vi "GUI_Bella_IP2_plasma1.vi"() -> ()   [LabVIEW 2020]
uses:
  Shared/GUI_Template/GUI_master/tcp_new_data_event.ctl
  Shared/GUI_Template/GUI_master/tcp new data cluster.ctl
  Device Drivers/FilterWheels/posTypDef.ctl
  <vilib>/vision/Image Controls.llb/IMAQ Image.ctl
panel:
  in  "GUIdevice 21":string="FW-PL1-General"
  in  "pos.Channel4::21":T1=enum."4" caption="dpm cam"
  in  "Position.Axis 1::9":dbl=0.00011 caption="DPM - Y" min=-200.0 max=200.0 format="%.3g"
  in  "Boolean":bool
  out "String":string="off"
  in  "position::20":dbl=0.049403 caption="DPM_aligncam" min=0.0 max=50.0 format="%.3g"
  in  "trigger::1":bool caption="Trigger"
  in  "trigger::2":bool caption="Trigger"
  in  "exposure::2":dbl=0.005 caption="exposure" min=3.8e-05 max=1.0 format="%.3p"
  in  "Target.X::2":dbl=200.0 caption="X" min=0.0 max=2000.0
  in  "Target.Y::2":dbl=200.0 caption="Y" min=0.0 max=2000.0
  in  "TargetSize.X::2":dbl=50.0 caption="Size X" min=2.0 max=3000.0
  in  "Color 2":u32(colorbox)=16711680 caption="Color"
  in  "TargetSize.Y::2":dbl=50.0 caption="Size Y" min=2.0 max=3000.0
  in  "Thickness 2":u8=3
  out "SideViewNorth":T2(plugin-control)
  in  "exposure::1":dbl=0.001 caption="exposure" min=3.8e-05 max=1.0 format="%.3p"
  out "DPM_Align_IP2":T2(plugin-control)
  in  "Target.X::1":dbl=838.0 caption="X" min=0.0 max=2000.0
  in  "Target.Y::1":dbl=620.0 caption="Y" min=0.0 max=2000.0
  in  "TargetSize.X::1":dbl=50.0 caption="Size X" min=2.0 max=3000.0
  in  "Color 1":u32(colorbox)=16711680 caption="Color"
  in  "TargetSize.Y::1":dbl=50.0 caption="Size Y" min=2.0 max=3000.0
  in  "Thickness 1":u8=3
  in  "GUIdevice 2":string="CAM-PL1-SideviewNorth" caption="GUIdevice 4"
  out "image::2":T2(plugin-control) caption="M1 Cam"
  out "image::1":T2(plugin-control) caption="M1 Cam"
  in  "GUIdevice 1":string="CAM-PL1-DPM_Align_IP2" caption="GUIdevice 4"
  in  "position::20":dbl=0.049403 caption="DPM_aligncam" min=0.0 max=50.0 format="%.3g"
  in  "GUIdevice 20":string="STAGE-PL1-LPmodeLong"
  in  "Position.Axis 3::8":dbl=70000.0 caption="Pico Btm \nHrz" min=-1000000.0 max=1000000.0 format="%.3g"
  in  "Position.Axis 2::9":dbl=0.00011 caption="IP2 SMF" min=0.0 max=25.0 format="%.3g"
  in  "Position.Axis 3::9":dbl=47.0 caption="Debris Shield" min=-200.0 max=200.0 format="%.3g"
  in  "GUIdevice 9":string="MCD-PL1-ESP301-1" caption="GUIdevice 4"
  in  "Position.Stage B::19":dbl=57.000013 caption="DPM - Y" min=-200.0 max=200.0 format="%.3g"
  in  "Position.Stage C::18":dbl=-36.99999 caption="DPM - Z" min=-100.0 max=100.0 format="%.3g"
  in  "Position.Stage A::18":dbl=165.499987 caption="DPM - X" min=-400.0 max=400.0 format="%.3g"
  in  "GUIdevice 19":string="MCD-PL1-NewmarkDPMY"
  in  "GUIdevice 18":string="MCD-PL1-NewmarkDPMXZ"
  in  "Position.Axis 4::8":dbl=25400.0 caption="Pico Btm \nVert" min=-100000.0 max=100000.0 format="%.3g"
  in  "Position.Axis 2::8":dbl=200.0 caption="Pico Top \nHrz" min=-100000.0 max=100000.0 format="%.3g"
  in  "Position.Axis 1::8":dbl=-8000.0 caption="Pico Top \nVert" min=-100000.0 max=100000.0 format="%.3g"
  in  "GUIdevice 8":string="MCD-PL1-picosOFI1" caption="GUIdevice 4"
  out "tcp data event":T3
  in  "stop":bool
  out "error IO 2":errorcluster
  # "Plasma 1 + M3"
  # "DPM Alignment"
  # "DPM Major Axes, Picos, Debris Shield"
  # "<----laser"
  # "Filter Wheels"
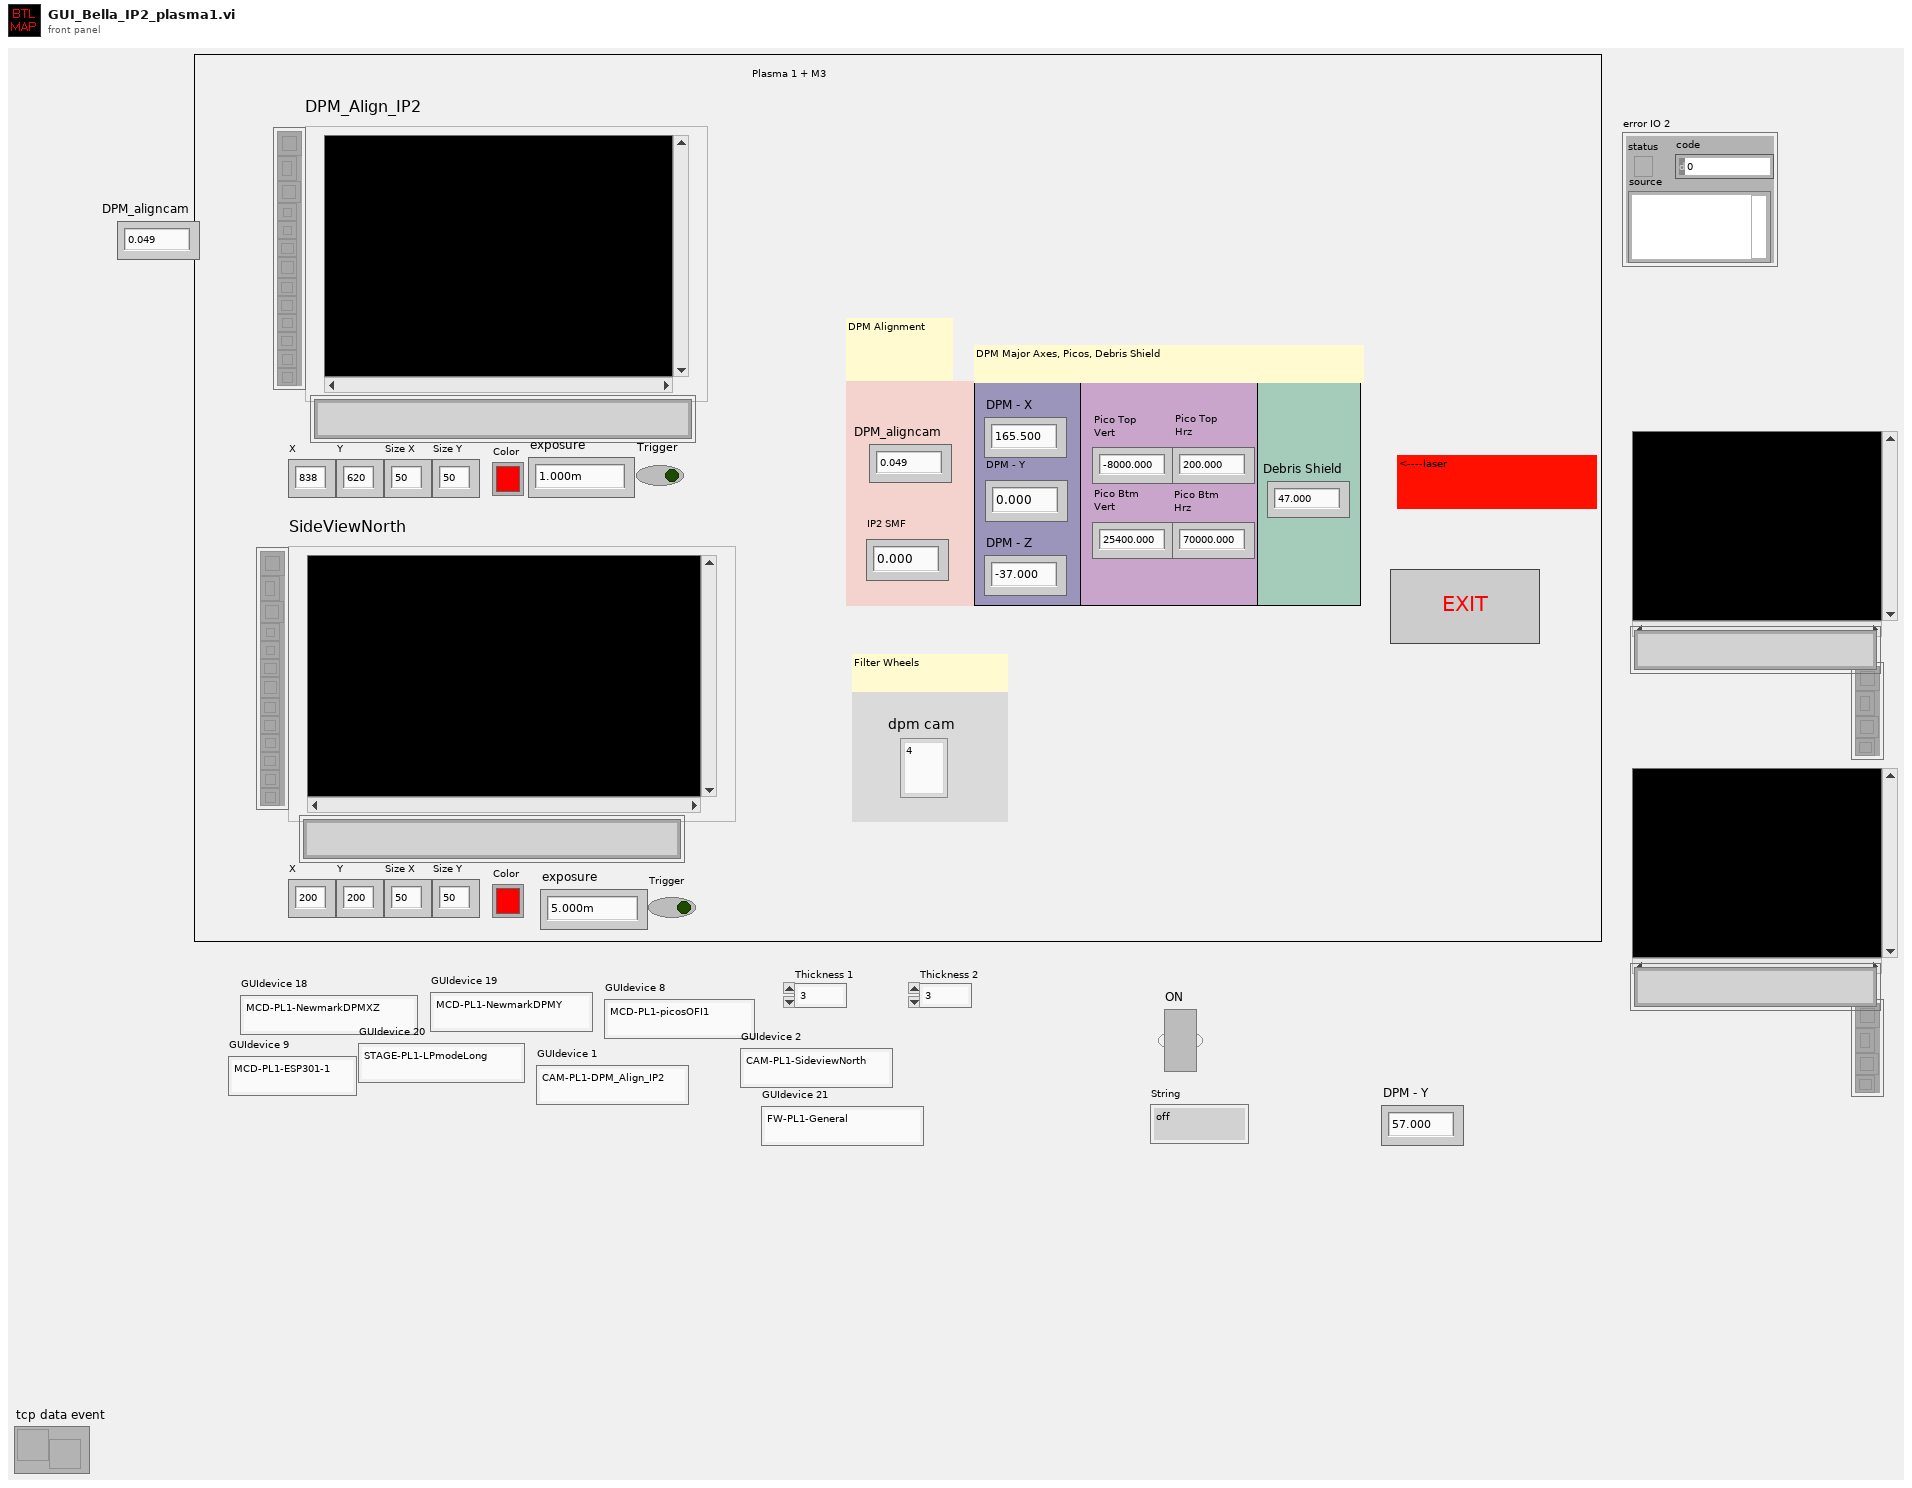
[diagram p1: front panel]
types:
  T1 = typedef "posTypDef.ctl" = enum16{"1", "2", "3", "4", "5", "6"}
  T2 = typedef "IMAQ Image.ctl" = refnum<image>
  T3 = typedef "tcp_new_data_event.ctl" = refnum<user-event>
  T4 = cluster{"Last update Cam1":u32, "Last update Cam2":u32, "Last update Cam3":u32, "Last update Cam4":u32, "Last update Cam5":u32, "Last update Cam6":u32, "Last update Cam7":u32, "Last update Cam8":u32}
  T5 = typedef "Image Type" = u32
  T6 = typedef "tcp new data cluster.ctl" = cluster{"EventEnum":enum16{"new data", "connection status update"}, "Device name":string}
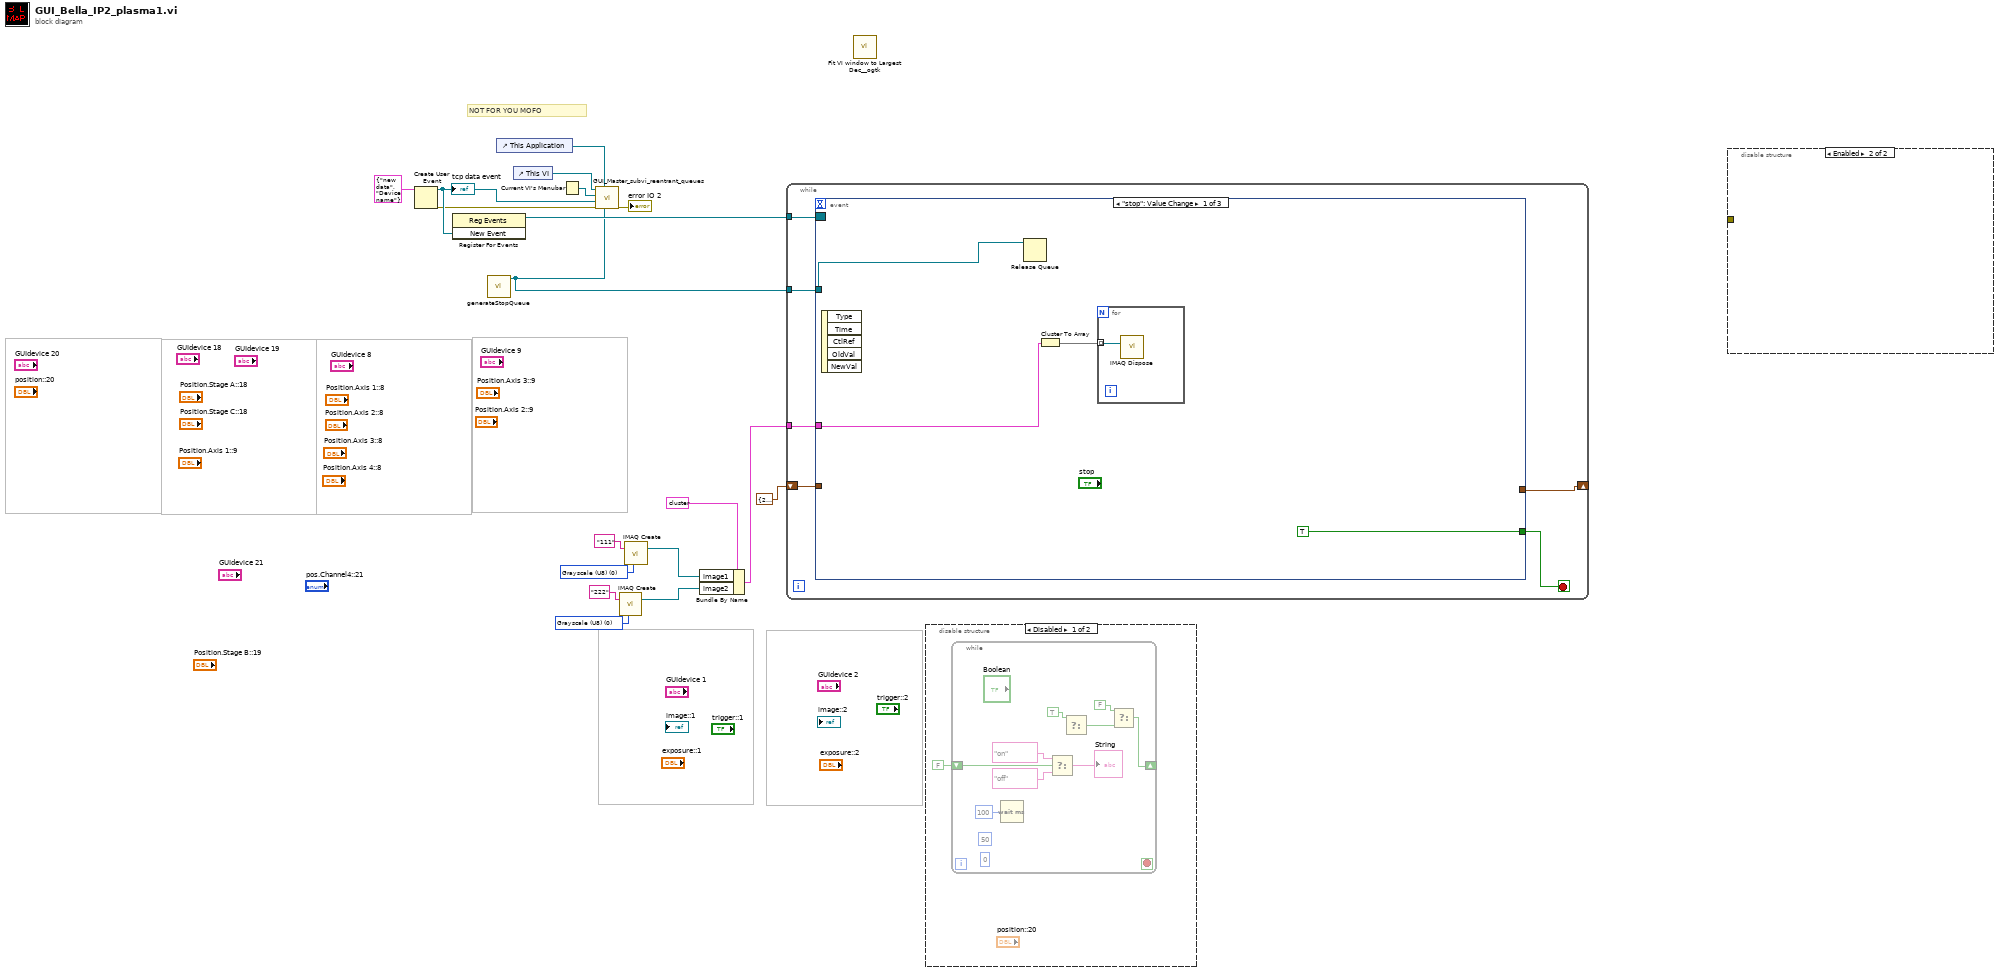
[diagram p0: block diagram]
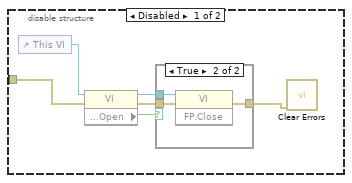
[diagram p3: hidden frame]
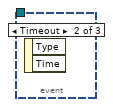
[diagram p5: hidden frame]
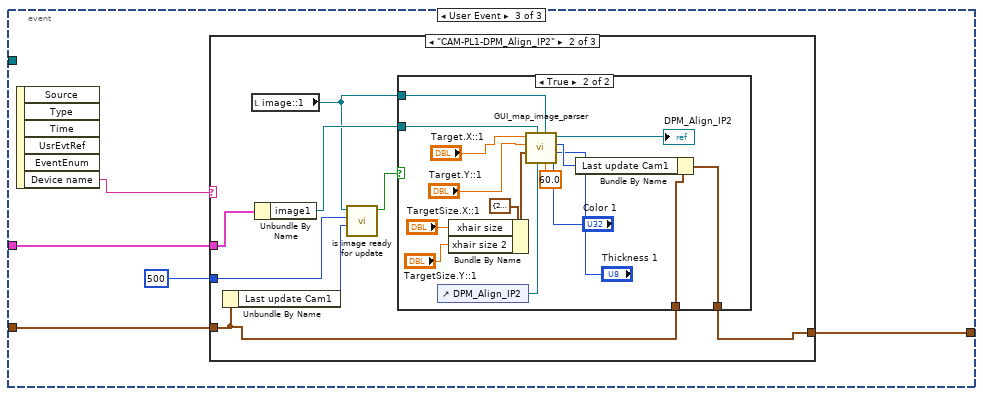
[diagram p6: hidden frame]
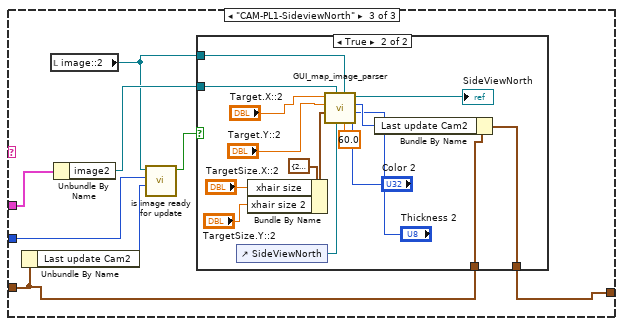
[diagram p9: hidden frame]
diagram:
  w8 = T5 0 items=["Grayscale (U8)", "Grayscale (I16)", "Grayscale (SGL)", "Complex (CSG)", "RGB (U32)", "HSL (U32)", "RGB (U64)", "Grayscale (U16)"] ("Image Type")
  w10 = T5 0 items=["Grayscale (U8)", "Grayscale (I16)", "Grayscale (SGL)", "Complex (CSG)", "RGB (U32)", "HSL (U32)", "RGB (U64)", "Grayscale (U16)"] ("Image Type")
  # "NOT FOR YOU MOFO"
  n1 = Create User Event(user event datatype=T6 {"EventEnum"=enum."new data", "Device name"="Device name"} ("New Event")) -> (user event=w17:refnum<user-event>, error out=w16:errorcluster)  [unwired: 1 in]
  "tcp data event" <- w17
  n2 = register-events(w17) -> (reference out=w11:refnum<event-registration>)  [unwired: 2 in, 1 out]
  n3 = call "generateStopQueue.vi"() -> ("STOP Queue out"=w1:refnum<queue>)  [unwired: 10 in, 1 out]
  n4 = control-ref of="This Application"() -> (w18:refnum<vi>)
  n5 = control-ref of="This VI"() -> (w13:refnum<vi>)
  n6 = Current VI's Menubar() -> (w14:refnum<k9>)
  n7 = call "GUI_Master_subvi_reentrant_queues.vi"("STOP Queue in"=w1, "This Application"=w18, "error in (no error)"=w16, "tcp data event"=w17, "Caller menu reference"=w14, "Caller VI ref"=w13) -> ("error out"=→"error IO 2":errorcluster)  [unwired: 5 in]
  n8 = call "IMAQ Create"("Image Name"="222", "Image Type"=w10) -> ("New Image"=w5:T2)  [unwired: 3 in, 1 out]
  n9 = call "IMAQ Create"("Image Name"="111", "Image Type"=w8) -> ("New Image"=w6:T2)  [unwired: 3 in, 1 out]
  n10 = Bundle By Name(cluster=cluster{"image1":T2, "image2":T2} {"image1"="image1", "image2"="image2"} ("input cluster"), "image1"=w6, "image2"=w5) -> (w3:cluster{"image1":T2, "image2":T2})
  n11 = while {
    tunnel: w11 -> [w23]
    tunnel: w3 -> [w22]
    shift-right: [w20] -> _
    shift-left: T4 {"Last update Cam1"=200, "Last update Cam2"=200, "Last update Cam3"=200, "Last update Cam4"=200, "Last update Cam5"=200, "Last update Cam6"=200, "Last update Cam7"=200, "Last update Cam8"=200} -> [w21]
    tunnel: w1 -> [w19]
    stop <- w24 stop-if-true
    n12 = event shown="[0] \"stop\": Value Change" {
      selector: w23 -> [_ _ _]
      dyn-events: _ -> [_ _ _]
      timeout: _ -> [_ _ _]
      tunnel: [TRUE ("stop") _ _] -> w24
      tunnel: w22 -> [w25 _ w33]
      tunnel: w21 -> [_ _ w32]
      tunnel: [_ _ w31] -> w20
      tunnel: w19 -> [w27 _ _]
      event "stop": Value Change {
        n13 = event-data() -> ()  [unwired: 1 in, 5 out]
        n14 = Release Queue(queue=w27) -> ()  [unwired: 2 in, 3 out]
        n15 = Cluster To Array(cluster=w25) -> (array=w26:T2[])
        n16 = for {
          tunnel: w26 -> [w29] mode=indexing
          n17 = call "IMAQ Dispose"("Image"=w29) -> ()  [unwired: 5 in, 1 out]
        }
      }
      event Timeout {
        n18 = event-data() -> ()  [unwired: 1 in, 2 out]
      }
      event User Event {
        n19 = event-data() -> ("Device name"=w34:string)  [unwired: 1 in, 5 out]
        n20 = case shown="\"CAM-PL1-DPM_Align_IP2\"" w34 {
          tunnel: w33 -> [_ w39 w64]
          tunnel: w32 -> [w35 w41 w66]
          tunnel: [w35 w40 w65] -> w31
          tunnel: u32 500 ("x-y") -> [_ w36 w61]
          frame "False", Default {
          }
          frame "CAM-PL1-DPM_Align_IP2" {
            n21 = Unbundle By Name(w41) -> ("Last update Cam1"=w42:u32)
            n22 = local read "image::1"() -> (w37:T2)
            n23 = Unbundle By Name(w39) -> ("image1"=w38:T2)
            n24 = call "is image ready for update.vi"("Last update"=w42, "min time between updates"=w36, "image ref in"=w37) -> ("update image"=w43:bool)  [unwired: 8 in]
            n25 = case shown="True" w43 {
              tunnel: w41 -> [w44 w60]
              tunnel: [w44 w59] -> w40
              tunnel: w37 -> [_ w58]
              tunnel: w38 -> [_ w50]
              frame False {
              }
              frame True {
                n26 = control-ref of="DPM_Align_IP2"() -> (w45:refnum<vi>)
                n27 = Bundle By Name(cluster=cluster{"xhair size":dbl, "xhair size 2":dbl} {"xhair size"=20.0, "xhair size 2"=20.0} ("size"), "xhair size"="TargetSize.X::1", "xhair size 2"="TargetSize.Y::1") -> (w51:cluster{"xhair size":dbl, "xhair size 2":dbl})
                n28 = call "GUI_map_image_parser.vi"("color"="Color 1", "Thickness"="Thickness 1", "zoom#"=60.0, "Image Src"=w58, "Ctl Refnum"=w45, "Image Dst"=w50, "size"=w51, "target y"="Target.Y::1", "target x"="Target.X::1") -> ("ms timer out"=w55:u32, "Img out"=→"DPM_Align_IP2":T2)  [unwired: 1 in]
                n29 = Bundle By Name(cluster=w60, "Last update Cam1"=w55) -> (w59:T4)
              }
            }
          }
          frame "CAM-PL1-SideviewNorth" {
            n30 = Unbundle By Name(w66) -> ("Last update Cam2"=w67:u32)
            n31 = local read "image::2"() -> (w62:T2)
            n32 = Unbundle By Name(w64) -> ("image2"=w63:T2)
            n33 = call "is image ready for update.vi"("Last update"=w67, "min time between updates"=w61, "image ref in"=w62) -> ("update image"=w68:bool)  [unwired: 8 in]
            n34 = case shown="True" w68 {
              tunnel: w66 -> [w69 w85]
              tunnel: [w69 w84] -> w65
              tunnel: w62 -> [_ w83]
              tunnel: w63 -> [_ w75]
              frame False {
              }
              frame True {
                n35 = control-ref of="SideViewNorth"() -> (w70:refnum<vi>)
                n36 = Bundle By Name(cluster=cluster{"xhair size":dbl, "xhair size 2":dbl} {"xhair size"=20.0, "xhair size 2"=20.0} ("size"), "xhair size"="TargetSize.X::2", "xhair size 2"="TargetSize.Y::2") -> (w76:cluster{"xhair size":dbl, "xhair size 2":dbl})
                n37 = call "GUI_map_image_parser.vi"("color"="Color 2", "Thickness"="Thickness 2", "zoom#"=60.0, "Image Src"=w83, "Ctl Refnum"=w70, "Image Dst"=w75, "size"=w76, "target y"="Target.Y::2", "target x"="Target.X::2") -> ("ms timer out"=w80:u32, "Img out"=→"SideViewNorth":T2)  [unwired: 1 in]
                n38 = Bundle By Name(cluster=w85, "Last update Cam2"=w80) -> (w84:T4)
              }
            }
          }
        }
      }
    }
  }
  n39 = call <userlib>:"Fit VI window to Largest Dec__ogtk.vi"() -> ()  [unwired: 6 in, 2 out]
  n40 = disable-structure shown="Disabled" {
    frame Disabled {
      n41 = while {
        shift-right: [w92] -> _
        shift-left: FALSE -> [w90]
        stop <- _ stop-if-true
        (unwired) 0
        (unwired) 50
        n42 = Wait (ms)(milliseconds to wait=u32 100 ("millisecond timer value")) -> ()  [unwired: 1 out]
        n43 = Select(t="on", s=w90, f="off") -> (s? t:f=→"String":string)
        n44 = Select(t=TRUE) -> (s? t:f=w91:bool)  [unwired: 2 in]
        n45 = Select(t=FALSE, f=w91) -> (s? t:f=w92:bool)  [unwired: 1 in]
      }
    }
    frame Enabled {
    }
  }
  n46 = disable-structure shown="Enabled" {
    disable-tunnel: _ -> [w97 _]
    frame Disabled {
      n47 = control-ref of="This VI"() -> (w98:refnum<vi>)
      n48 = property class="VI"(reference=w98, error in=w97) -> (reference out=w100:refnum<vi>, error out=w101:errorcluster, "Front Panel.Open"=w99:bool)
      n49 = case shown="True" w99 {
        tunnel: [w102 w105] -> w96
        tunnel: w101 -> [w102 w104]
        tunnel: w100 -> [_ w103]
        frame False {
        }
        frame True {
          n50 = invoke class="VI" method="FP.Close"(reference=w103, error in=w104) -> (error out=w105:errorcluster)  [unwired: 1 in, 2 out]
        }
      }
      n51 = call <vilib>:"Clear Errors.vi"("error in (no error)"=w96) -> ()  [unwired: 5 in, 2 out]
    }
    frame Enabled {
    }
  }
